vi "test Receive Signal.vi"(11 "Test Case In":refnum<class "Test PCAN.lvclass">) -> (0 "error out":errorcluster, 3 "Test Case Out":refnum<class "Test PCAN.lvclass">)   [LabVIEW 2024, in "Test PCAN.lvclass"]
uses:
  Test PCAN.lvclass
  C:/Program Files/National Instruments/LabVIEW 2024/vi.lib/Astemes/LUnit/Test Case.lvclass
  PCAN.lvclass
  D:/git/HAL/HAL/Configurations/CFG JSON/CFG JSON.lvclass
  Configurations/CFG JSON/CFG JSON.lvclass
  D:/git/HAL/HAL/Configurations/CFG Base/CFG Base.lvclass
  Protocols/ICAN/ICAN.lvclass
  Configurations/CFG Base/CFG Base.lvclass/CFG Base.ctl
  <vilib>/Astemes/LUnit/Test Case.lvclass/Test Case.ctl
  <vilib>/JDP Science/JSONtext/Next JSON Value.vi
  <vilib>/JDP Science/JSONtext/String Subset.vi
  <vilib>/Astemes/LUnit/Append Pass Result.vi
  <vilib>/Astemes/LUnit/Append Fail Result.vi
  <vilib>/JDP Science/JSONtext/Parsing/Advance past next JSON Value (inlined COPY).vi
  <vilib>/Astemes/LUnit/Run In UI.vi
  <vilib>/JDP Science/JSONtext/Parsing/Advance past whitespace.vi
  <vilib>/JDP Science/JSONtext/Parsing/Advance past String.vi
  <vilib>/JDP Science/JSONtext/Parsing/Advance past Number.vi
  <vilib>/Utility/error.llb/Clear Errors.vi
  <vilib>/JDP Science/JSONtext/Parsing/Advance past Line Ending.vi
  <vilib>/JDP Science/JSONtext/Parsing/Parse Full Path or Item Name.vi
  <vilib>/JDP Science/JSONtext/Parsing/Advance past Array.vi
  <vilib>/JDP Science/JSONtext/Parsing/Advance past Object.vi
  <vilib>/JDP Science/JSONtext/support/Error Cluster From Code.vi
  <vilib>/JDP Science/JSONtext/Offset/Find Item Locations by Path.vi
  <vilib>/Astemes/LUnit/Test Case.lvclass
  <vilib>/JDP Science/JSONtext/JSONtext.lvlib
  Configurations/CFG Base/CFG Base.lvclass
panel:
  out "Output":variant
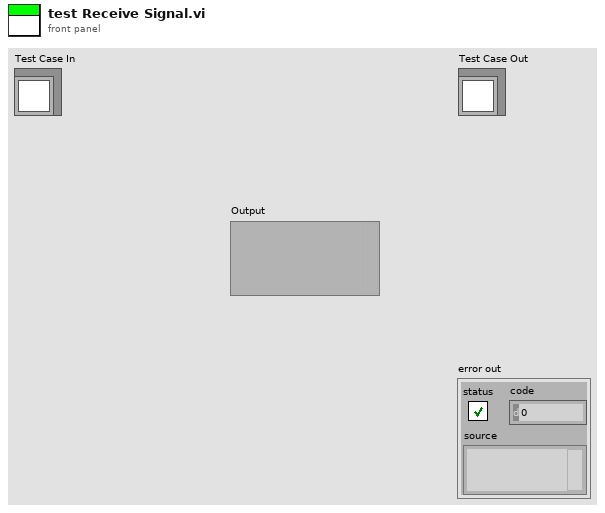
[diagram p1: front panel]
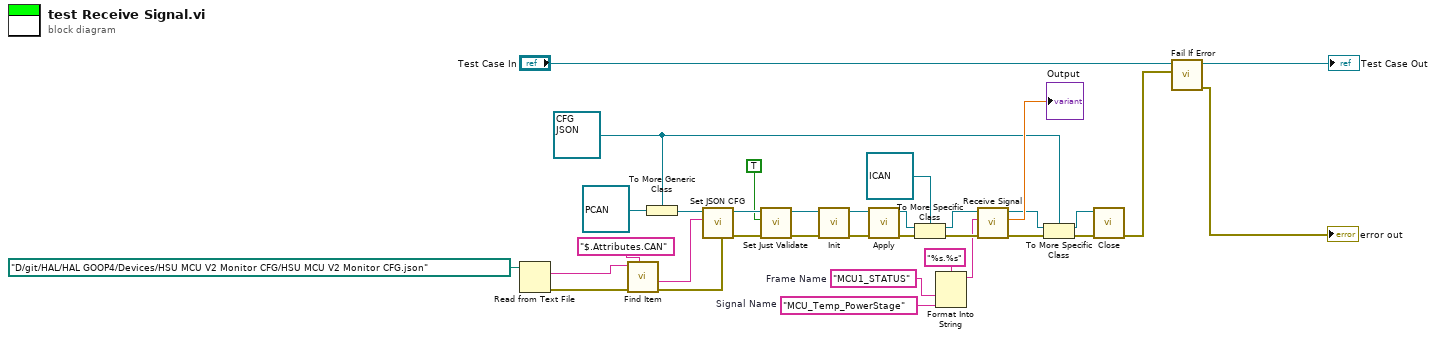
[diagram p0: block diagram]
diagram:
  w7 = "MCU1_STATUS"  # Frame Name
  w6 = "MCU_Temp_PowerStage"  # Signal Name
  w13 = refnum<class "CFG JSON.lvclass"> refnum ("HAL GOOP4.lvlib:CFG JSON.lvclass")
  n1 = Read from Text File(file (use dialog)=path "D:/git/HAL/HAL GOOP4/Devices/HSU MCU V2 Monitor CFG/HSU MCU V2 Monitor CFG.json") -> (text=w4:string, error out=w21:errorcluster)  [unwired: 3 in, 2 out]
  n2 = call <vilib>:"Find Item.vi"("$Path or Item Name"="$.Attributes.CAN", "error in (no error)"=w21, "JSON"=w4) -> ("error out"=w1:errorcluster, "<JSON>"=w3:string)  [unwired: 5 in, 2 out]
  n3 = To More Generic Class(target class=w13, reference=refnum<class "PCAN.lvclass"> refnum ("PCAN.lvclass")) -> (generic class reference=w28:refnum<class "CFG JSON.lvclass">)
  n4 = call "Set JSON CFG.vi"("<JSON> CFG"=w3, "CFG JSON in"=w28) -> ("CFG JSON out"=w27:refnum<class "CFG JSON.lvclass">)  [unwired: 9 in]
  n5 = call "Set Just Validate.vi"("Just Validate"=TRUE, "CFG Base in"=w27) -> ("CFG Base out"=w25:refnum<class "CFG JSON.lvclass">)  [unwired: 9 in]
  n6 = call-dynamic "Init.vi"("error in"=w1, "CFG Base in"=w25) -> ("error out"=w26:errorcluster, "CFG Base out"=w23:refnum<class "CFG JSON.lvclass">)  [unwired: 8 in]
  n7 = call-dynamic "Apply.vi"("error in"=w26, "CFG Base in"=w23) -> ("error out"=w20:errorcluster, "CFG Base out"=w18:refnum<class "CFG JSON.lvclass">)  [unwired: 8 in]
  n8 = To More Specific Class(target class=refnum<class "ICAN.lvclass"> refnum ("ICAN.lvclass"), reference=w18, error in=w20) -> (specific class reference=w16:refnum<class "ICAN.lvclass">, error out=w19:errorcluster)
  n9 = Format Into String(format string="%s.%s", w7, w6) -> (resulting string=w5:string)  [unwired: 2 in, 1 out]
  n10 = call-dynamic "Receive Signal.vi"("error in"=w19, "Frame.Signal"=w5, "ICommunicate in"=w16) -> ("error out"=w12:errorcluster, "Value"=→"Output":dbl, "ICommunicate out"=w10:refnum<class "ICAN.lvclass">)  [unwired: 6 in]
  n11 = To More Specific Class(target class=w13, reference=w10, error in=w12) -> (specific class reference=w9:refnum<class "CFG JSON.lvclass">, error out=w11:errorcluster)
  n12 = call-dynamic "Close.vi"("error in"=w11, "CFG Base in"=w9) -> ("error out"=w14:errorcluster)  [unwired: 8 in, 1 out]
  n13 = call <vilib>:"Fail If Error.vi"("Assert error"=w14, "LUnit Test Case In"="Test Case In") -> ("error out"=→"error out":errorcluster, "LUnit Test Case Out"=→"Test Case Out":refnum<class "Test PCAN.lvclass">)  [unwired: 8 in]
